vi "FindValue.vi"(8 "键":string="d", 11 "键值串":string="[a=a][b=b][c=c]") -> (0 "值":string, 3 "存在?":bool)   [LabVIEW 2020, in "Curve Editor.lvlib" / "Key Value.lvlib"]
uses:
  Key Value.lvlib
panel:
  # "从键值串中查询键的值，并返回查询结果"
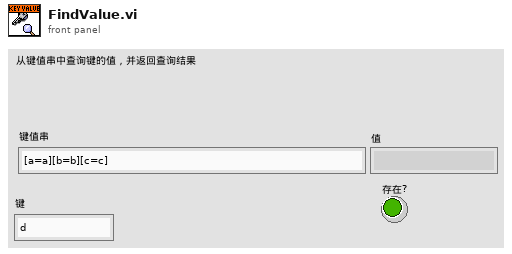
[diagram p1: front panel]
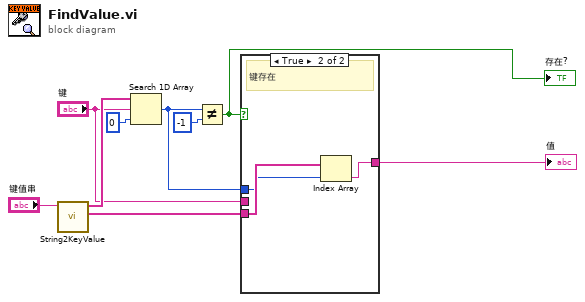
[diagram p0: block diagram]
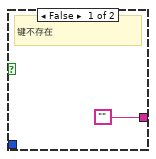
[diagram p2: hidden frame]
diagram:
  n1 = call "String2KeyValue.vi"("健值对字符串"="键值串") -> ("值数组"=w5:string[], "键数组"=w3:string[])  [unwired: 9 in]
  n2 = Search 1D Array(1D array=w3, element="键", start index (0)=0 ("开始索引(0)")) -> (index of element=w4:i32)
  n3 = Not Equal?(x=w4, y=-1) -> (x != y?=w6:bool)
  "存在?" <- w6
  n4 = case shown="True" w6 {
    tunnel: w5 -> [_ w13]
    tunnel: w4 -> [_ w12]
    tunnel: "键" -> [_ _]
    tunnel: ["" w11] -> w1
    frame False {
      # "键不存在"
    }
    frame True {
      # "键存在"
      n5 = Index Array(array=w13, index=w12) -> (element=w11:string)
    }
  }
  "值" <- w1
